vi "get_single_acq.vi"(8 "error in (no error)":errorcluster, 11 "dummyCam in":refnum<class "dummyCam.lvclass">) -> (0 "error out":errorcluster, 1 "wavelength":dbl[](array[numeric]), 2 "intensity":dbl[][](array[numeric]), 3 "dummyCam out":refnum<class "dummyCam.lvclass">, 4 "trig channel 2":bool[](array[boolean]), 6 "trig channel 1":bool[](array[boolean]))   [LabVIEW 2018, in "dummyCam.lvclass"]
uses:
  dummyCam.lvclass
  globals/current_timestep.vi
  globals/current_t0.vi
  _cameraBase/_cameraBase.lvclass
  <vilib>/Analysis/NI_AALBase.lvlib
  <vilib>/gmath/NI_Gmath.lvlib
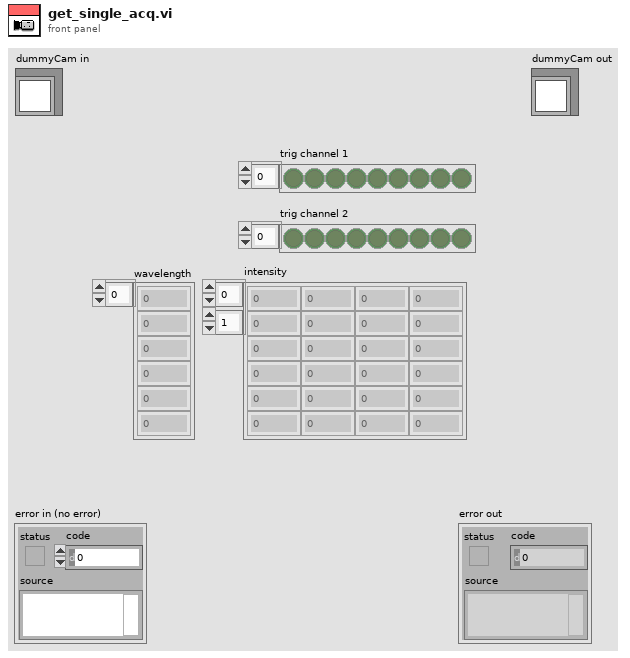
[diagram p1: front panel]
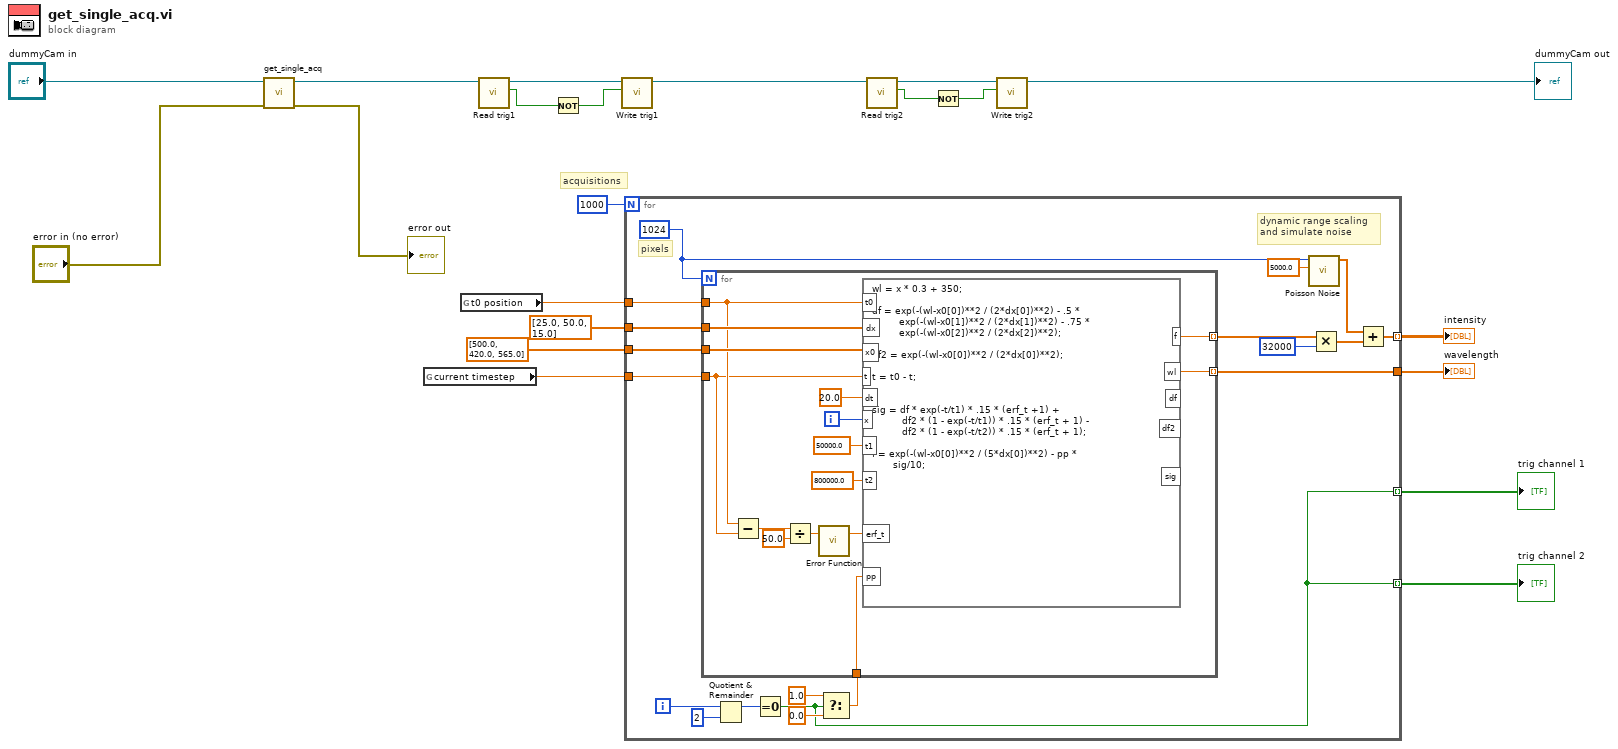
[diagram p0: block diagram]
diagram:
  # "acquisitions"
  n1 = call-parent "get_single_acq.vi"("error in (no error)"="error in (no error)", "_cameraBase in"="dummyCam in") -> ("error out"=→"error out":errorcluster, "_cameraBase out"=w11:refnum<class "dummyCam.lvclass">)  [unwired: 4 in, 4 out]
  n2 = global read "current_timestep.vi" "current timestep"() -> (w15:dbl)
  n3 = global read "current_t0.vi" "t0 position"() -> (w12:dbl)
  n4 = call-dynamic "Read trig1.vi"("_cameraBase in"=w11) -> ("trig1"=w4:bool, "_cameraBase out"=w10:refnum<class "dummyCam.lvclass">)  [unwired: 8 in, 1 out]
  n5 = Not(x=w4) -> (.not. x?=w3:bool)
  n6 = call-dynamic "Write trig1.vi"("trig1"=w3, "_cameraBase in"=w10) -> ("_cameraBase out"=w9:refnum<class "dummyCam.lvclass">)  [unwired: 8 in, 1 out]
  n7 = for {
    N: 1000 -> [_]
    tunnel: [w33] -> w18 mode=indexing
    tunnel: [w35] -> w17
    tunnel: w15 -> [w26]
    tunnel: w12 -> [w25]
    tunnel: dbl[] [500.0, 420.0, 565.0] -> [w24]
    tunnel: dbl[] [25.0, 50.0, 15.0] -> [w23]
    tunnel: [w22] -> w2 mode=indexing
    tunnel: [w22] -> w1 mode=indexing
    i -> [w28]
    w39 = 1024
    # "pixels"
    # "dynamic range scaling\nand simulate noise"
    n8 = Quotient & Remainder(x=w28, y=2) -> (x-y*floor(x/y)=w32:i32)  [unwired: 1 out]
    n9 = Equal To 0?(x=w32) -> (x = 0?=w22:bool)
    n10 = Select(t=1.0, s=w22, f=0.0) -> (s? t:f=w27:dbl)
    n11 = for {
      N: w39 -> [_]
      tunnel: [w55] -> w37 mode=indexing
      tunnel: [w54] -> w35 mode=indexing
      tunnel: w27 -> [w46]
      tunnel: w26 -> [w41]
      tunnel: w25 -> [w42]
      tunnel: w24 -> [w45]
      tunnel: w23 -> [w44]
      i -> [w47]
      n12 = Subtract(x=w42, y=w41) -> (x-y=w50:dbl)
      n13 = Divide(x=w50, y=50.0) -> (x/y=w49:dbl)
      n14 = call <vilib>:"Error Function.vi"("x"=w49) -> ("erf(x)"=w51:dbl)  [unwired: 2 in]
      n15 = formula code="wl = x * 0.3 + 350;\n\ndf = exp(-(wl-x0[0])**2 / (2*dx[0])**2) - .5 *\n         exp(-(wl-x0[1])**2 / (2*dx[1])**2) - .75 * \n         exp(-(wl-x0[2])**2 / (2*dx[2])**2);\n\ndf2 = exp(-(wl-x0[0])**2 / (2*dx[0])**2);\n\nt = t0 - t;\n\n\nsig = df * exp(-t/t1) * .15 * (erf_t +1) +\n          df2 * (1 - exp(-t/t1)) * .15 * (erf_t + 1) -\n          df2 * (1 - exp(-t/t2)) * .15 * (erf_t + 1);\n\nf = exp(-(wl-x0[0])**2 / (5*dx[0])**2) - pp * \n       sig/10;"("x"=w47, "x0"=w45, "dx"=w44, "t"=w41, "dt"=20.0 ("input variable"), "t0"=w42, "t1"=50000.0 ("input variable"), "erf_t"=w51, "pp"=w46, "t2"=800000.0 ("input variable")) -> ("f"=w55:dbl, "wl"=w54:dbl)  [unwired: 3 out]
    }
    n16 = call <vilib>:"Poisson Noise.vi"("mean"=5000.0, "samples"=w39) -> ("poisson noise"=w38:dbl[])  [unwired: 8 in, 1 out]
    n17 = Multiply(x=w37, y=32000) -> (x*y=w34:dbl[])
    n18 = Add(x=w38, y=w34) -> (x+y=w33:dbl[])
  }
  "intensity" <- w18
  "wavelength" <- w17
  "trig channel 1" <- w2
  "trig channel 2" <- w1
  n19 = call-dynamic "Read trig2.vi"("_cameraBase in"=w9) -> ("trig2"=w6:bool, "_cameraBase out"=w8:refnum<class "dummyCam.lvclass">)  [unwired: 8 in, 1 out]
  n20 = Not(x=w6) -> (.not. x?=w5:bool)
  n21 = call-dynamic "Write trig2.vi"("trig2"=w5, "_cameraBase in"=w8) -> ("_cameraBase out"=→"dummyCam out":refnum<class "dummyCam.lvclass">)  [unwired: 8 in, 1 out]
